vi "dfd_Simplify LM Factors.vi"(8 "M_in":i32, 11 "L_in":i32) -> (0 "M_out":i32, 3 "L_out":i32, 4 "relPrime?":bool)   [LabVIEW 2017, in "NI_DigFilterLicensed.lvlib"]
uses:
  <vilib>/addons/Digital Filter Design/NI_DigFilterLicensed.lvlib
  <vilib>/gmath/NI_Gmath.lvlib
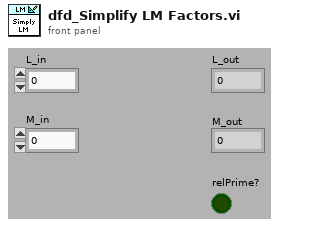
[diagram p1: front panel]
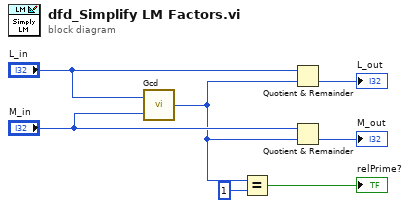
[diagram p0: block diagram]
diagram:
  n1 = call <vilib>:"Gcd.vi"("y"="M_in", "x"="L_in") -> ("gcd(x,y)"=w3:i32)
  n2 = Equal?(x=w3, y=1) -> (x = y?=→"relPrime?":bool)
  n3 = Quotient & Remainder(x="L_in", y=w3) -> (floor(x/y)=→"L_out":i32)  [unwired: 1 out]
  n4 = Quotient & Remainder(x="M_in", y=w3) -> (floor(x/y)=→"M_out":i32)  [unwired: 1 out]
